vi "Read Internal Temperature.vi"(8 "error in (no error)":errorcluster, 11 "VISA resource name":refnum<visa-resource-name>) -> (0 "error out":errorcluster, 2 "Internal Temperature":dbl, 3 "VISA resource name out":refnum<visa-resource-name>)   [LabVIEW 2019, in "Keithley 2182.lvlib"]
doc: "Reads the instrument's internal temperature."
uses:
  Keithley 2182.lvlib
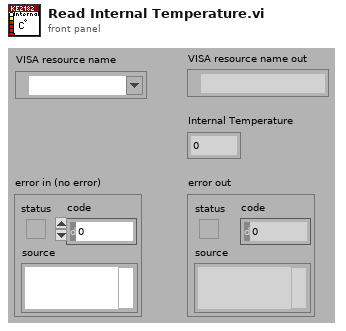
[diagram p1: front panel]
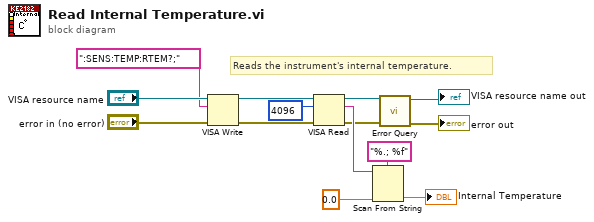
[diagram p0: block diagram]
diagram:
  # "Reads the instrument's internal temperature."
  n1 = VISA Write(VISA resource name="VISA resource name", write buffer=":SENS:TEMP:RTEM?;" ("command"), error in (no error)="error in (no error)") -> (VISA resource name out=w6:refnum<visa-resource-name>, error out=w5:errorcluster)  [unwired: 1 out]
  n2 = VISA Read(VISA resource name=w6, byte count=u32 4096, error in (no error)=w5) -> (VISA resource name out=w2:refnum<visa-resource-name>, read buffer=w11:string, error out=w3:errorcluster)  [unwired: 1 out]
  n3 = Scan From String(format string="%.; %f", input string=w11, default 1=0.0 ("default value 1")) -> (output 1=→"Internal Temperature":dbl)  [unwired: 2 in, 3 out]
  n4 = call "Error Query.vi"("error in (no error)"=w3, "VISA resource name"=w2) -> ("error out"=→"error out":errorcluster, "VISA resource name out"=→"VISA resource name out":refnum<visa-resource-name>)  [unwired: 6 in, 2 out]
